vi "CE14.open handshake(subVI).vi"(8 "error in(no error)":errorcluster, 11 "VISA resource name":refnum<visa-resource-name>) -> (0 "error out":errorcluster, 1 "success":bool, 2 "response msg":string[](array[string]), 3 "VISA resource name 2":refnum<visa-resource-name>)   [LabVIEW 2018, in "CE14_eMIC.lvlib"]
uses:
  CE14_eMIC.lvlib
  type defs/CE14_state.ctl
  <vilib>/Instr/_visa.llb/VISA Configure Serial Port (Instr).vi
  <vilib>/Utility/error.llb/Error Cluster From Error Code.vi
  <vilib>/ErrorRing/Error Ring.xnode
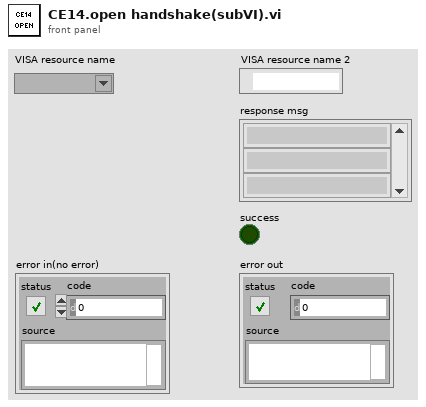
[diagram p1: front panel]
types:
  T1 = typedef "CE14_eMIC.lvlib/CE14_state.ctl" = enum16{"open COM (300)", "step1(300):2F 3F 21 0D 0A", "step2(300):06 30 34 31 0D 0A", "step3:Change4800", "step4(4800)", "stop"}
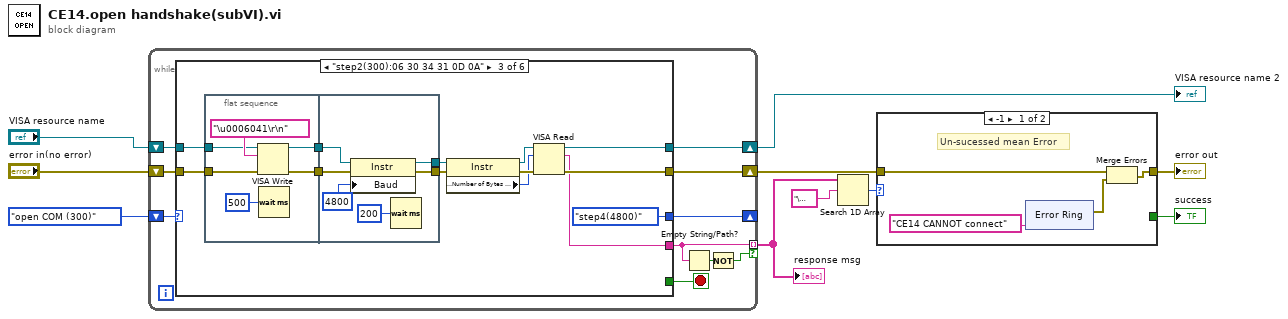
[diagram p0: block diagram]
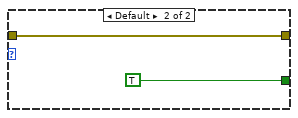
[diagram p2: hidden frame]
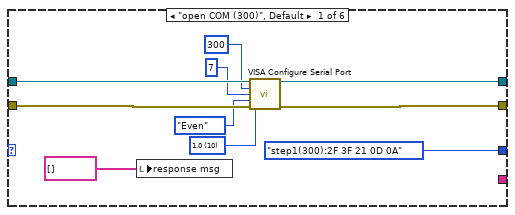
[diagram p3: hidden frame]
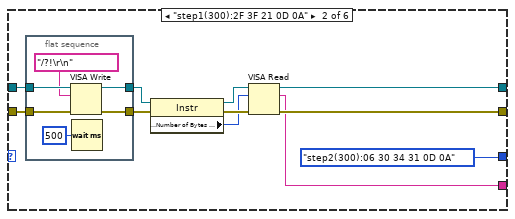
[diagram p4: hidden frame]
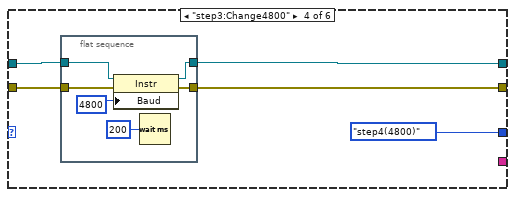
[diagram p5: hidden frame]
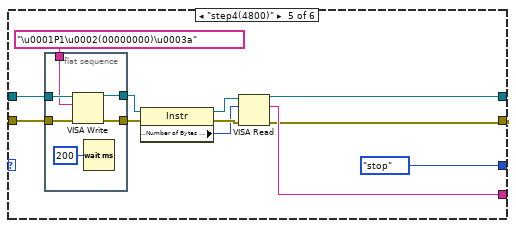
[diagram p6: hidden frame]
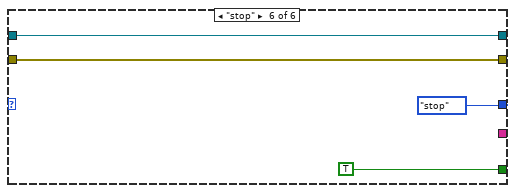
[diagram p7: hidden frame]
diagram:
  n1 = while {
    shift-right: [w19] -> w5
    shift-left: "VISA resource name" -> [w20]
    shift-right: [w18] -> w7
    shift-left: "error in(no error)" -> [w17]
    tunnel: [w15] -> w4 mode=indexing if=w11
    shift-right: [w14] -> _
    shift-left: CE14_state."open COM (300)" -> [w12]
    stop <- w13 stop-if-true
    n2 = case shown="\"step2(300):06 30 34 31 0D 0A\"" w12 {
      tunnel: w20 -> [w26 w41 w59 w77 w93 w104]
      tunnel: [w30 w34 w52 w74 w86 w104] -> w19
      tunnel: [w27 w36 w54 w75 w85 w103] -> w18
      tunnel: w17 -> [w25 w40 w60 w76 w92 w103]
      tunnel: [_ w32 w50 _ w94 _] -> w15
      tunnel: [CE14_state."step1(300):2F 3F 21 0D 0A" CE14_state."step2(300):06 30 34 31 0D 0A" CE14_state."step4(4800)" CE14_state."step4(4800)" CE14_state."stop" CE14_state."stop"] -> w14
      tunnel: [_ _ _ _ _ TRUE] -> w13
      frame "open COM (300)", Default {
        w21 = u16 10 items=["1.0"=10, "1.5"=15, "2.0"=20] ("stop bits (10: 1 bit)")
        n3 = local write "response msg"(string[] []) -> ()
        n4 = call-poly "VISA Configure Serial Port"("VISA resource name"=w26, "baud rate (9600)"=u32 300, "data bits (8)"=u16 7, "parity (0:none)"=enum16{"None", "Odd", "Even", "Mark", "Space"}."Even", "error in (no error)"=w25, "stop bits (10: 1 bit)"=w21) -> ("VISA resource name out"=w30:refnum<visa-resource-name>, "error out"=w27:errorcluster)  [unwired: 8 in]
      }
      frame "step1(300):2F 3F 21 0D 0A" {
        n5 = flat-sequence {
          tunnel: w41 -> [w47]
          tunnel: w40 -> [w46]
          tunnel: [w45] -> w39
          tunnel: [w44] -> w38
          frame #0 {
            n6 = VISA Write(VISA resource name=w47, write buffer="/?!\r\n", error in (no error)=w46) -> (VISA resource name out=w44:refnum<visa-resource-name>, error out=w45:errorcluster)  [unwired: 1 out]
            n7 = Wait (ms)(milliseconds to wait=u32 500) -> ()  [unwired: 1 out]
          }
        }
        n8 = property class="Instr"(reference=w38, error in=w39) -> (reference out=w35:refnum<visa-resource-name>, error out=w37:errorcluster, "Serial Settings:Number of Bytes at Serial Port"=w33:u32)
        n9 = VISA Read(VISA resource name=w35, byte count=w33, error in (no error)=w37) -> (VISA resource name out=w34:refnum<visa-resource-name>, read buffer=w32:string, error out=w36:errorcluster)  [unwired: 1 out]
      }
      frame "step2(300):06 30 34 31 0D 0A" {
        n10 = flat-sequence {
          tunnel: w59 -> [w62]
          tunnel: w60 -> [w61]
          tunnel: [w64] -> w49
          tunnel: [w63] -> w48
          tunnel: w49 -> [w69]
          tunnel: w48 -> [w68]
          tunnel: [w71] -> w57
          tunnel: [w70] -> w55
          frame #0 {
            n11 = VISA Write(VISA resource name=w62, write buffer="\u0006041\r\n", error in (no error)=w61) -> (VISA resource name out=w63:refnum<visa-resource-name>, error out=w64:errorcluster)  [unwired: 1 out]
            n12 = Wait (ms)(milliseconds to wait=u32 500) -> ()  [unwired: 1 out]
          }
          frame #1 {
            n13 = property class="Instr"(reference=w68, error in=w69, "Baud"=u32 4800 ("Serial Settings:Baud Rate")) -> (reference out=w70:refnum<visa-resource-name>, error out=w71:errorcluster)
            n14 = Wait (ms)(milliseconds to wait=u32 200) -> ()  [unwired: 1 out]
          }
        }
        n15 = property class="Instr"(reference=w55, error in=w57) -> (reference out=w53:refnum<visa-resource-name>, error out=w56:errorcluster, "Serial Settings:Number of Bytes at Serial Port"=w51:u32)
        n16 = VISA Read(VISA resource name=w53, byte count=w51, error in (no error)=w56) -> (VISA resource name out=w52:refnum<visa-resource-name>, read buffer=w50:string, error out=w54:errorcluster)  [unwired: 1 out]
      }
      frame "step3:Change4800" {
        n17 = flat-sequence {
          tunnel: w77 -> [w82]
          tunnel: w76 -> [w81]
          tunnel: [w80] -> w75
          tunnel: [w79] -> w74
          frame #0 {
            n18 = property class="Instr"(reference=w82, error in=w81, "Baud"=u32 4800 ("Serial Settings:Baud Rate")) -> (reference out=w79:refnum<visa-resource-name>, error out=w80:errorcluster)
            n19 = Wait (ms)(milliseconds to wait=u32 200) -> ()  [unwired: 1 out]
          }
        }
      }
      frame "step4(4800)" {
        n20 = flat-sequence {
          tunnel: w93 -> [w99]
          tunnel: w92 -> [w98]
          tunnel: "\u0001P1\u0002(00000000)\u0003a" ("write buffer") -> [w97]
          tunnel: [w101] -> w91
          tunnel: [w100] -> w88
          frame #0 {
            n21 = VISA Write(VISA resource name=w99, write buffer=w97, error in (no error)=w98) -> (VISA resource name out=w100:refnum<visa-resource-name>, error out=w101:errorcluster)  [unwired: 1 out]
            n22 = Wait (ms)(milliseconds to wait=u32 200) -> ()  [unwired: 1 out]
          }
        }
        n23 = property class="Instr"(reference=w88, error in=w91) -> (reference out=w89:refnum<visa-resource-name>, error out=w90:errorcluster, "Serial Settings:Number of Bytes at Serial Port"=w87:u32)
        n24 = VISA Read(VISA resource name=w89, byte count=w87, error in (no error)=w90) -> (VISA resource name out=w86:refnum<visa-resource-name>, read buffer=w94:string, error out=w85:errorcluster)  [unwired: 1 out]
      }
      frame "stop" {
      }
    }
    n25 = Empty String/Path?(string/path=w15) -> (empty?=w16:bool)
    n26 = Not(x=w16) -> (.not. x?=w11:bool)
  }
  "response msg" <- w4
  "VISA resource name 2" <- w5
  n27 = Search 1D Array(1D array=w4, element="\u0006") -> (index of element=w2:i32)  [unwired: 1 in]
  n28 = case shown="-1" w2 {
    tunnel: w7 -> [w108 w118]
    tunnel: [w106 w118] -> w6
    tunnel: [_ TRUE] -> w1
    frame -1 {
      # "Un-sucessed mean Error"
      n29 = xnode ("Error Ring")("parameter 0"="CE14 CANNOT connect") -> ("error out"=w107:errorcluster)
      n30 = Merge Errors(w108, w107) -> (w106:errorcluster)
    }
    frame Default {
    }
  }
  "error out" <- w6
  "success" <- w1
